vi "Calculator.vi"() -> ()   [LabVIEW 2019]
panel:
  in  "Stop Button":bool
  out "Display":string
  in  "Buttuns":T1
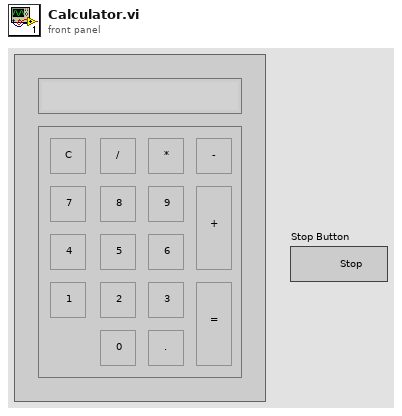
[diagram p1: front panel]
types:
  T1 = cluster{"Sub":bool, "Equal":bool, "dot":bool, "zero":bool, "three":bool, "two":bool, "one":bool, "six":bool, "five":bool, "four":bool, "nine":bool, "eight":bool, "seven":bool, "Sum":bool, "Mul":bool, "Div":bool, "Clear":bool}
  T2 = enum16{"Clear function", "Sum", "Sub", "Mul", "Div"}
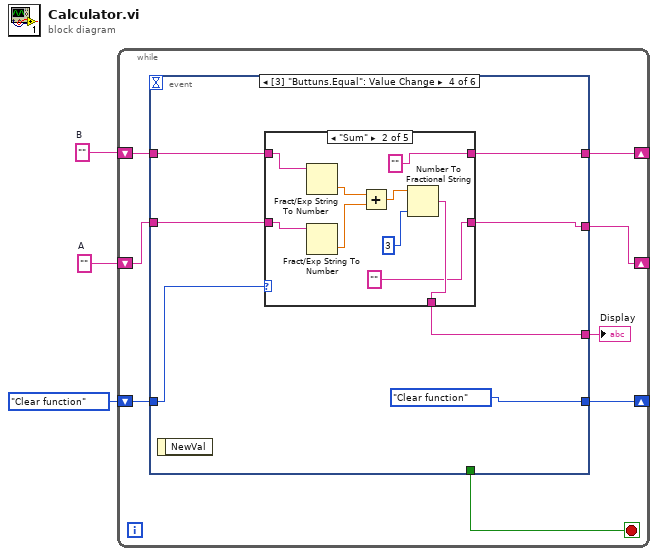
[diagram p0: block diagram]
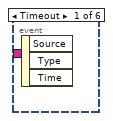
[diagram p2: hidden frame]
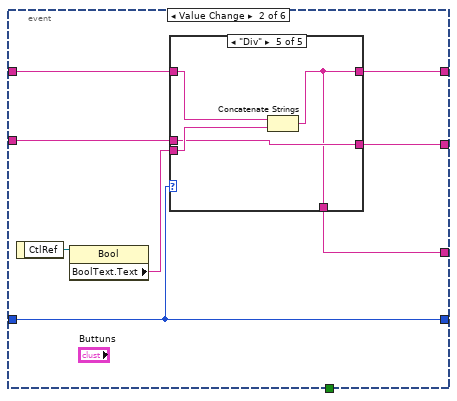
[diagram p3: hidden frame]
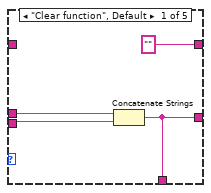
[diagram p4: hidden frame]
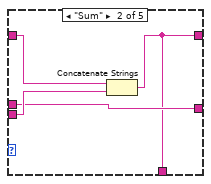
[diagram p5: hidden frame]
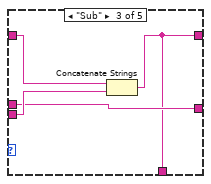
[diagram p6: hidden frame]
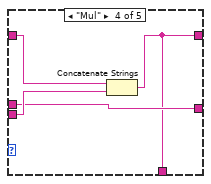
[diagram p7: hidden frame]
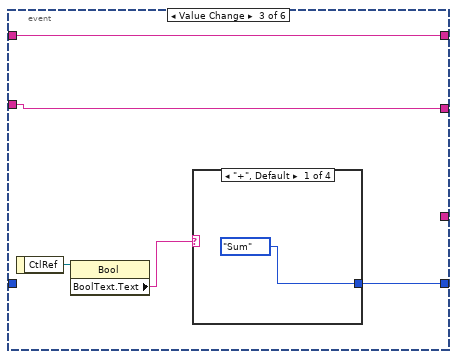
[diagram p8: hidden frame]
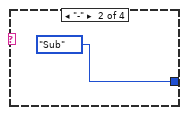
[diagram p9: hidden frame]
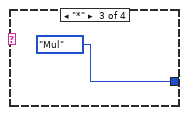
[diagram p10: hidden frame]
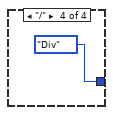
[diagram p11: hidden frame]
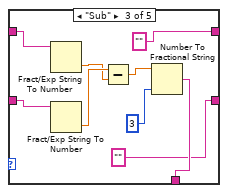
[diagram p13: hidden frame]
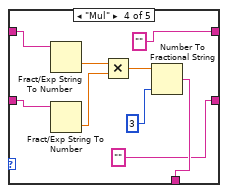
[diagram p14: hidden frame]
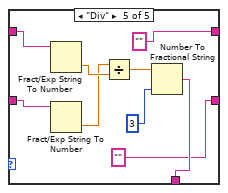
[diagram p15: hidden frame]
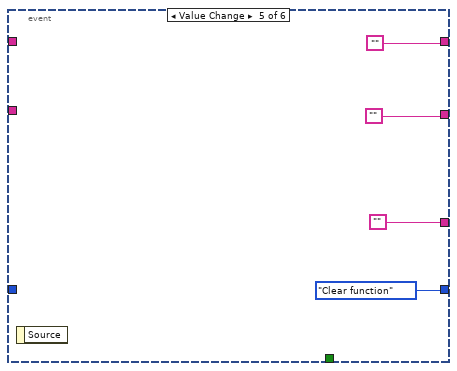
[diagram p16: hidden frame]
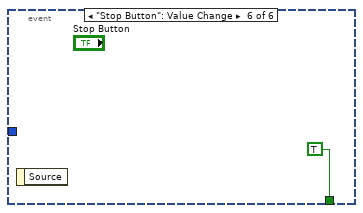
[diagram p17: hidden frame]
diagram:
  w3 = ""  # B
  w2 = ""  # A
  n1 = while {
    shift-right: [w5] -> _
    shift-left: w3 -> [w6]
    shift-right: [w8] -> _
    shift-left: w2 -> [w9]
    shift-right: [w11] -> _
    shift-left: T2."Clear function" -> [w10]
    stop <- w4 stop-if-true
    n2 = event shown="[3] \"Buttuns.Equal\": Value Change" {
      selector: _ -> [_ _ _ _ _ _]
      dyn-events: _ -> [_ _ _ _ _ _]
      timeout: _ -> [_ _ _ _ _ _]
      tunnel: [_ w19 w42 T2."Clear function" T2."Clear function" _] -> w11
      tunnel: w10 -> [_ w19 _ w55 _ _]
      tunnel: w9 -> [_ w18 w40 w52 _ _]
      tunnel: [_ w15 w40 w53 "" _] -> w8
      tunnel: [_ w14 _ w49 "" _] -> w7
      tunnel: w6 -> [_ w13 w41 w50 _ _]
      tunnel: [_ w12 w41 w51 "" _] -> w5
      tunnel: [_ _ _ _ _ TRUE] -> w4
      event Timeout {
        n3 = event-data() -> ()  [unwired: 1 in, 3 out]
      }
      event "Buttuns.zero", "Buttuns.one", "Buttuns.two", "Buttuns.three", "Buttuns.four", "Buttuns.five", "Buttuns.six", "Buttuns.seven", "Buttuns.eight", "Buttuns.nine", "Buttuns.dot": Value Change {
        n4 = event-data() -> ("CtlRef"=w17:refnum<vi>)  [unwired: 1 in]
        n5 = property class="Bool"(reference=w17) -> ("BoolText.Text"=w16:string)  [unwired: 1 in, 2 out]
        n6 = case shown="\"Div\"" w19 {
          tunnel: w18 -> [w23 w25 w29 w33 w37]
          tunnel: w16 -> [w22 w26 w30 w34 w38]
          tunnel: [w21 w25 w29 w33 w37] -> w15
          tunnel: [w21 w24 w28 w32 w36] -> w14
          tunnel: w13 -> [_ w27 w31 w35 w39]
          tunnel: ["" w24 w28 w32 w36] -> w12
          frame "Clear function", Default {
            n7 = Concatenate Strings(w23, w22) -> (w21:string)
          }
          frame "Sum" {
            n8 = Concatenate Strings(w27, w26) -> (w24:string)
          }
          frame "Sub" {
            n9 = Concatenate Strings(w31, w30) -> (w28:string)
          }
          frame "Mul" {
            n10 = Concatenate Strings(w35, w34) -> (w32:string)
          }
          frame "Div" {
            n11 = Concatenate Strings(w39, w38) -> (w36:string)
          }
        }
      }
      event "Buttuns.Sum", "Buttuns.Sub", "Buttuns.Mul", "Buttuns.Div": Value Change {
        n12 = event-data() -> ("CtlRef"=w44:refnum<vi>)  [unwired: 1 in]
        n13 = property class="Bool"(reference=w44) -> ("BoolText.Text"=w43:string)  [unwired: 1 in, 2 out]
        n14 = case shown="\"+\", Default" w43 {
          tunnel: [T2."Sum" T2."Sub" T2."Mul" T2."Div"] -> w42
          frame "+", Default {
          }
          frame "-" {
          }
          frame "*" {
          }
          frame "/" {
          }
        }
      }
      event "Buttuns.Equal": Value Change {
        n15 = event-data() -> ()  [unwired: 1 in, 1 out]
        n16 = case shown="\"Sum\"" w55 {
          tunnel: [w56 "" "" "" ""] -> w53
          tunnel: w52 -> [w56 w62 w73 w82 w91]
          tunnel: [w57 "" "" "" ""] -> w51
          tunnel: w50 -> [w57 w63 w74 w83 w92]
          tunnel: [w56 w61 w72 w81 w90] -> w49
          frame "Clear function", Default {
          }
          frame "Sum" {
            n17 = Fract/Exp String To Number(string=w63) -> (number=w64:dbl)  [unwired: 3 in, 1 out]
            n18 = Fract/Exp String To Number(string=w62) -> (number=w65:dbl)  [unwired: 3 in, 1 out]
            n19 = Add(x=w64, y=w65) -> (x+y=w58:dbl)
            n20 = Number To Fractional String(number=w58, precision (6)=i16 3) -> (F-format string=w61:string)  [unwired: 2 in]
          }
          frame "Sub" {
            n21 = Fract/Exp String To Number(string=w74) -> (number=w68:dbl)  [unwired: 3 in, 1 out]
            n22 = Fract/Exp String To Number(string=w73) -> (number=w69:dbl)  [unwired: 3 in, 1 out]
            n23 = Subtract(x=w69, y=w68) -> (x-y=w67:dbl)
            n24 = Number To Fractional String(number=w67, precision (6)=i16 3) -> (F-format string=w72:string)  [unwired: 2 in]
          }
          frame "Mul" {
            n25 = Fract/Exp String To Number(string=w83) -> (number=w76:dbl)  [unwired: 3 in, 1 out]
            n26 = Fract/Exp String To Number(string=w82) -> (number=w77:dbl)  [unwired: 3 in, 1 out]
            n27 = Multiply(x=w76, y=w77) -> (x*y=w78:dbl)
            n28 = Number To Fractional String(number=w78, precision (6)=i16 3) -> (F-format string=w81:string)  [unwired: 2 in]
          }
          frame "Div" {
            n29 = Fract/Exp String To Number(string=w92) -> (number=w86:dbl)  [unwired: 3 in, 1 out]
            n30 = Fract/Exp String To Number(string=w91) -> (number=w85:dbl)  [unwired: 3 in, 1 out]
            n31 = Divide(x=w85, y=w86) -> (x/y=w87:dbl)
            n32 = Number To Fractional String(number=w87, precision (6)=i16 3) -> (F-format string=w90:string)  [unwired: 2 in]
          }
        }
      }
      event "Buttuns.Clear": Value Change {
        n33 = event-data() -> ()  [unwired: 1 in, 1 out]
      }
      event "Stop Button": Value Change {
        n34 = event-data() -> ()  [unwired: 1 in, 1 out]
      }
    }
    "Display" <- w7
  }
